vi "Get Byte Count Limit.vi"(8 "error in (no error)":errorcluster, 11 "RFFE Extended Command in":refnum<class "RFFE Extended Command.lvclass">) -> (0 "error out":errorcluster, 2 "Byte Count Limit":i32, 3 "RFFE Extended Command out":refnum<class "RFFE Extended Command.lvclass">)   [LabVIEW 2018, in "MIPI RFFE API.lvlib" / "RFFE Extended Command.lvclass"]
uses:
  RFFE Extended Command.lvclass
  Get Byte Count Field Width.vi
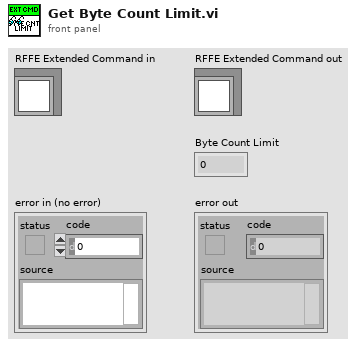
[diagram p1: front panel]
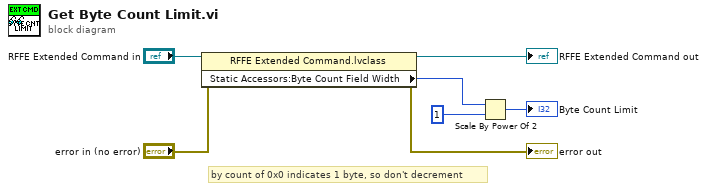
[diagram p0: block diagram]
diagram:
  # "by count of 0x0 indicates 1 byte, so don't decrement"
  n1 = property class="RFFE Extended Command.lvclass"(reference="RFFE Extended Command in", error in="error in (no error)") -> (reference out=→"RFFE Extended Command out":refnum<class "RFFE Extended Command.lvclass">, error out=→"error out":errorcluster, "Static Accessors:Byte Count Field Width"=w1:i32)
  n2 = Scale By Power Of 2(n=w1, x=1 ("Byte Count Limit")) -> (x*2^n=→"Byte Count Limit":i32)
